vi "pcfs_make_queues.vi"(8 "error in (no error)":errorcluster, 11 "pcfs in":refnum<class "pcfs.lvclass">) -> (0 "error out":errorcluster, 3 "pcfs out":refnum<class "pcfs.lvclass">)   [LabVIEW 2015, in "pcfs.lvclass"]
uses:
  pcfs.lvclass
  pcfs_loop_notifier_tdef.ctl
  pcfs.lvclass/pcfs.ctl
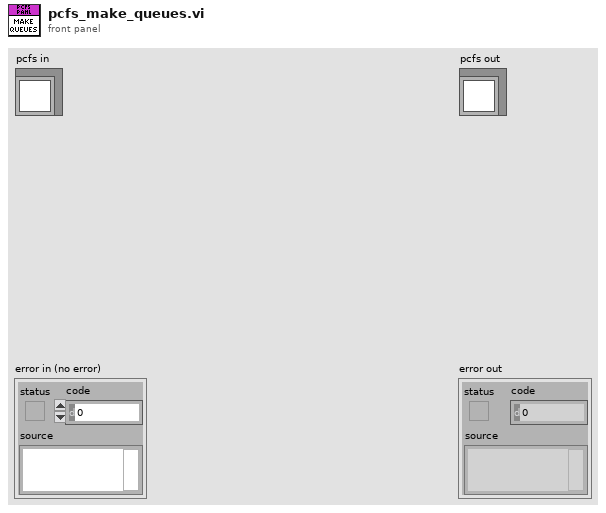
[diagram p1: front panel]
types:
  T1 = typedef "pcfs_loop_notifier_tdef.ctl" = enum16{"exit", "dither", "chart counts"}
  T2 = typedef "Rendezvous RefNum" = refnum<k1>
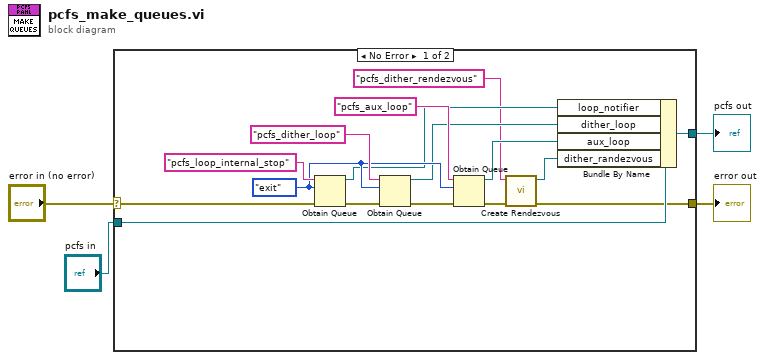
[diagram p0: block diagram]
diagram:
  n1 = case shown="No Error" "error in (no error)" {
    selector: "error in (no error)" -> [w20 w22]
    tunnel: [w5 w22] -> w3
    tunnel: [w10 w21] -> w1
    tunnel: "pcfs in" -> [w6 w21]
    frame No Error {
      w14 = pcfs_loop_notifier_tdef."exit" ("Enum")
      n2 = Obtain Queue(name (unnamed)="pcfs_loop_internal_stop", element data type=w14, error in (no error)=w20) -> (queue out=w13:refnum<queue>, error out=w18:errorcluster)  [unwired: 2 in, 1 out]
      n3 = Obtain Queue(name (unnamed)="pcfs_dither_loop", element data type=w14, error in (no error)=w18) -> (queue out=w12:refnum<queue>, error out=w16:errorcluster)  [unwired: 2 in, 1 out]
      n4 = Obtain Queue(name (unnamed)="pcfs_aux_loop", element data type=w14, error in (no error)=w16) -> (queue out=w11:refnum<queue>, error out=w9:errorcluster)  [unwired: 2 in, 1 out]
      n5 = call <vilib>:"Create Rendezvous.vi"("error in (no error)"=w9, "name (unnamed)"="pcfs_dither_rendezvous") -> ("error out"=w5:errorcluster, "rendezvous"=w7:T2)  [unwired: 3 in, 1 out]
      n6 = Bundle By Name(cluster=w6, "loop_notifier"=w13, "dither_loop"=w12, "aux_loop"=w11, "dither_randezvous"=w7) -> (w10:refnum<class "pcfs.lvclass">)
    }
    frame Error {
    }
  }
  "error out" <- w3
  "pcfs out" <- w1
